vi "my Poisson Random.vi"(6 "seed (-1)":i32=-1, 10 "lambda":dbl=1.0, 11 "samples (1)":i32=1) -> (0 "error":i32, 3 "Poisson random data":i32[](array[numeric]))   [LabVIEW 2021, in "Math.lvlib"]
uses:
  Math.lvlib
  <vilib>/gmath/statdist.llb/st_error_code.ctl
  <vilib>/gmath/statdist.llb/Uniform Random.vi
  <vilib>/gmath/NI_Gmath.lvlib
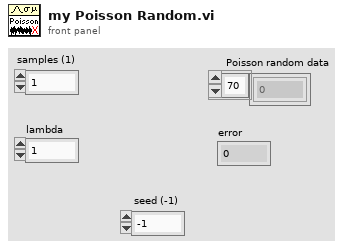
[diagram p1: front panel]
types:
  T1 = typedef "NI_Gmath.lvlib/st_error_code.ctl" = i32
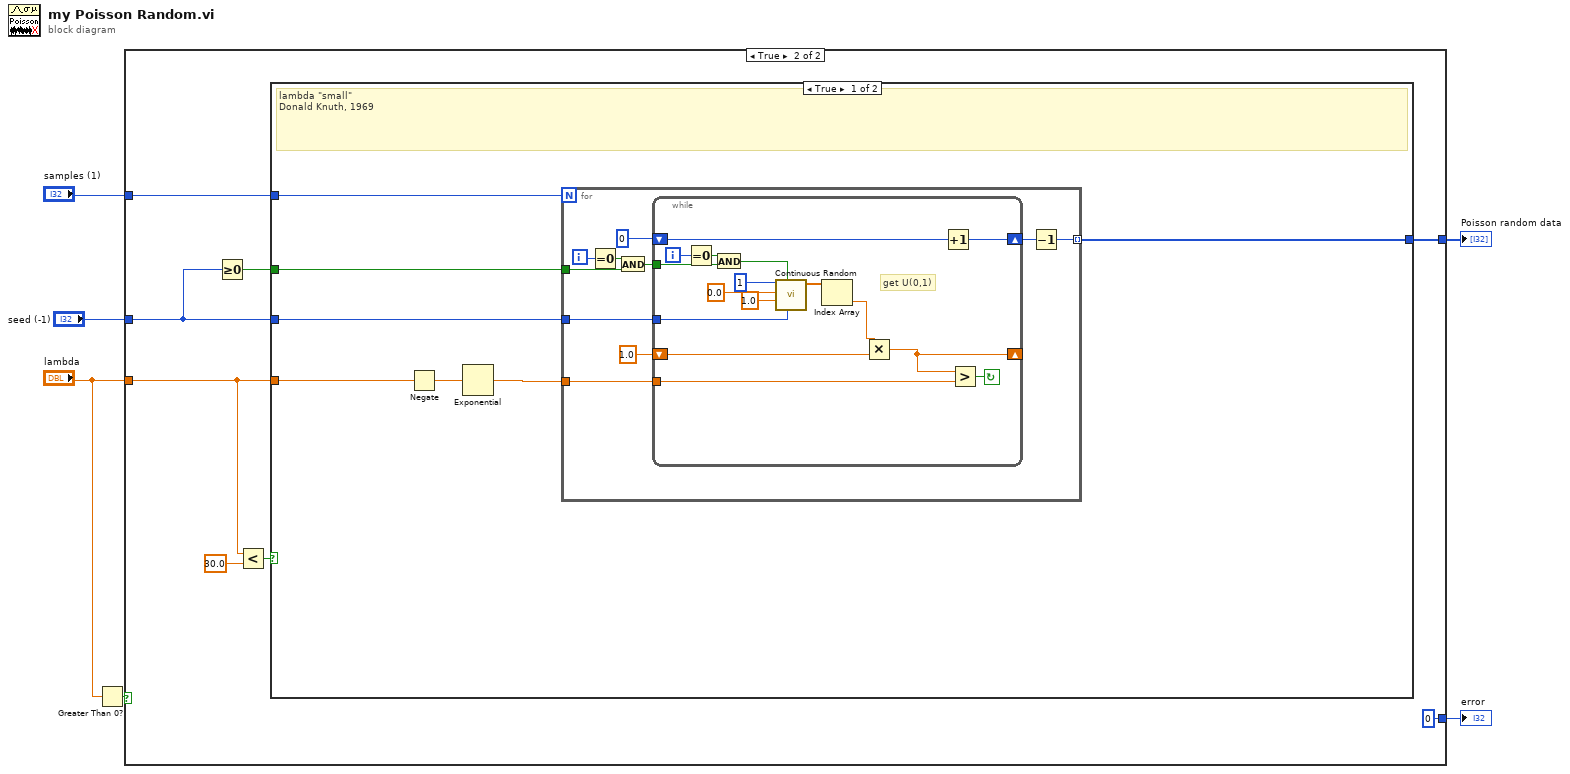
[diagram p0: block diagram]
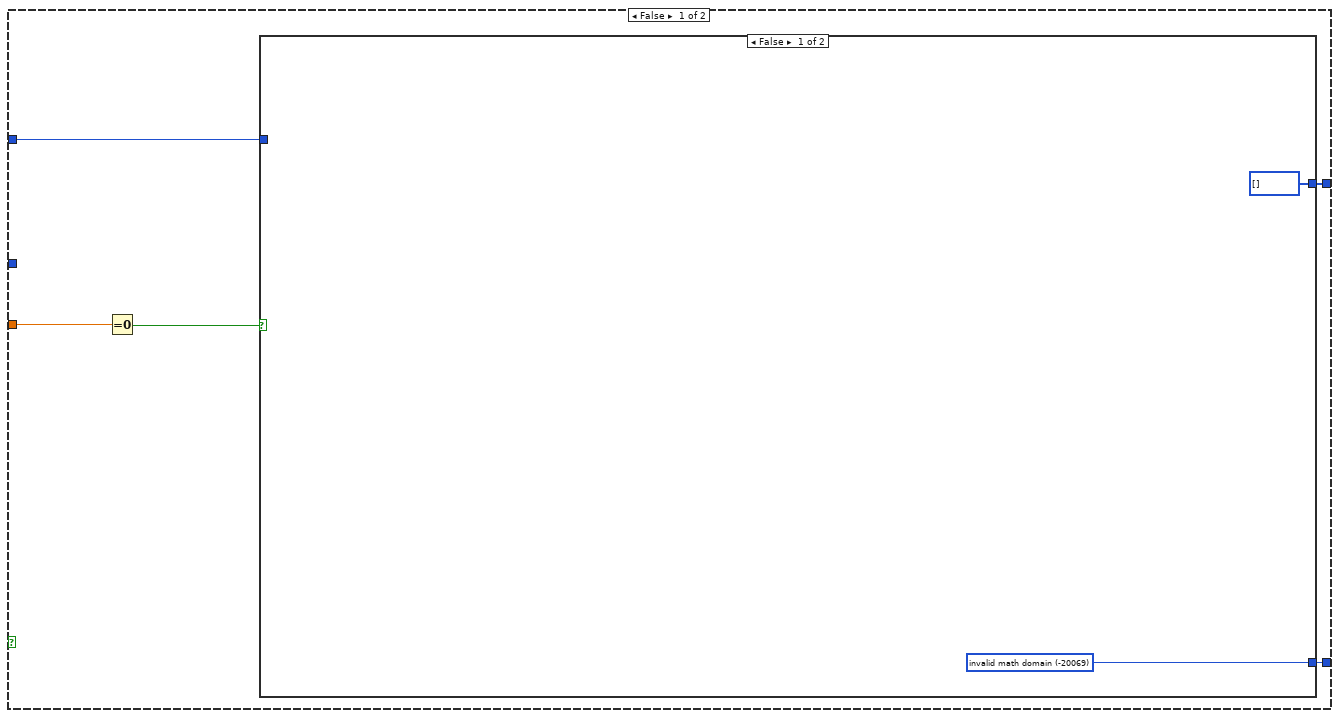
[diagram p2: hidden frame]
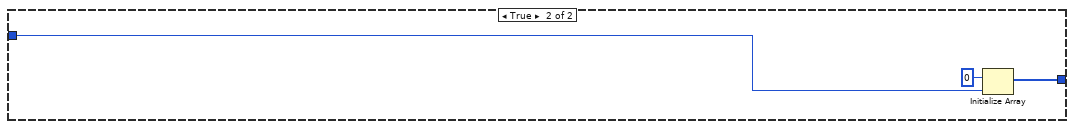
[diagram p3: hidden frame]
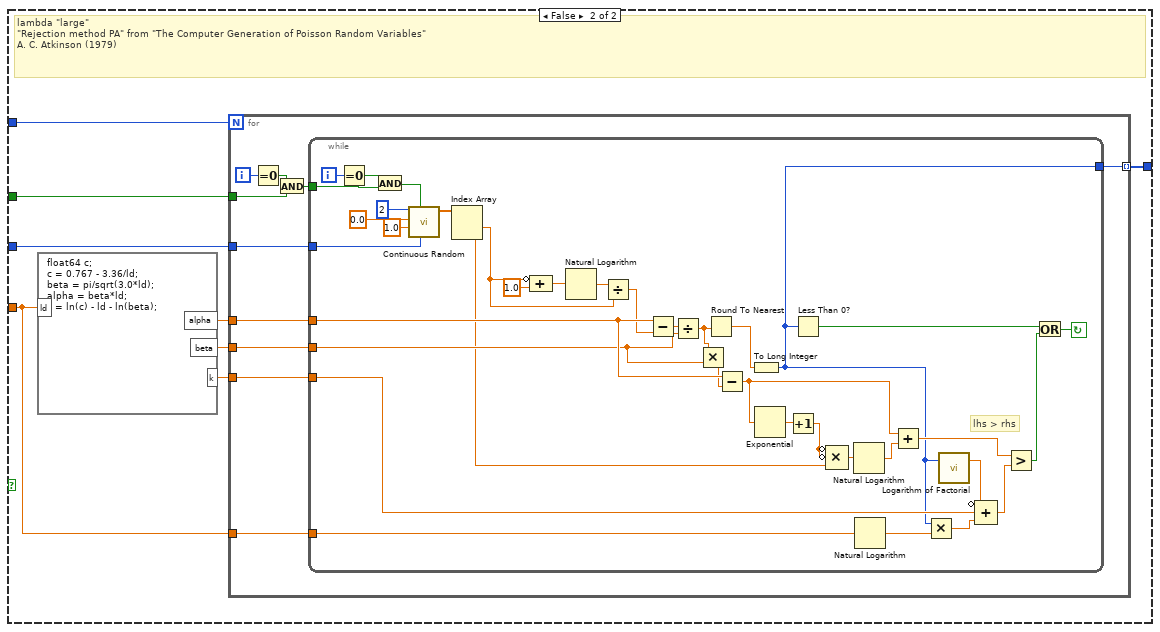
[diagram p4: hidden frame]
diagram:
  n1 = Greater Than 0?(x="lambda") -> (x > 0?=w6:bool)
  n2 = case shown="True" w6 {
    tunnel: [w11 w23] -> w3
    tunnel: "lambda" -> [w9 w19]
    tunnel: [w10 0 ("invalid math domain")] -> w2
    tunnel: "samples (1)" -> [w7 w22]
    tunnel: "seed (-1)" -> [_ w18]
    frame False {
      n3 = Equal To 0?(x=w9) -> (x = 0?=w8:bool)
      n4 = case shown="False" w8 {
        tunnel: [i32[] [] w16] -> w11
        tunnel: [w12 _] -> w10
        tunnel: w7 -> [_ w15]
        frame False {
          w12 = T1 -20069 items=["invalid math domain"=-20069, "Fourier interpolation size m >= n"=-20070, "empty array"=-20003] ("stat interp error code")
        }
        frame True {
          n5 = Initialize Array(0 ("element"), w15) -> (w16:i32[])
        }
      }
    }
    frame True {
      n6 = Greater Or Equal To 0?(x=w18) -> (x >= 0?=w17:bool)
      n7 = Less?(x=w19, y=30.0) -> (x < y?=w21:bool)
      n8 = case shown="True" w21 {
        tunnel: w19 -> [w31 w61]
        tunnel: [w28 w60] -> w23
        tunnel: w22 -> [w27 w65]
        tunnel: w18 -> [w26 w59]
        tunnel: w17 -> [w25 w58]
        frame True {
          # "lambda \"small\"\nDonald Knuth, 1969"
          n9 = Negate(x=w31) -> (-x=w30:dbl)
          n10 = Exponential(1:w30) -> (0:w29:dbl)
          n11 = for {
            N: w27 -> [_]
            tunnel: w29 -> [w40]
            tunnel: [w38] -> w28 mode=indexing
            tunnel: w26 -> [w36]
            tunnel: w25 -> [w34]
            i -> [w32]
            n12 = Equal To 0?(x=w32) -> (x = 0?=w35:bool)
            n13 = And(x=w35, y=w34) -> (x .and. y?=w33:bool)
            n14 = while {
              shift-right: [w56] -> w39
              shift-left: 0 -> [w57]
              tunnel: w40 -> [w55]
              shift-right: [w52] -> _
              shift-left: 1.0 -> [w53]
              tunnel: w36 -> [w46]
              tunnel: w33 -> [w44]
              i -> [w42]
              stop <- w54 continue-if-true
              # "get U(0,1)"
              n15 = Equal To 0?(x=w42) -> (x = 0?=w45:bool)
              n16 = And(x=w45, y=w44) -> (x .and. y?=w43:bool)
              n17 = call-poly <vilib>:"Continuous Random.vi"("seed"=w46, "reset"=w43, "xmax"=1.0, "xmin"=0.0, "samples"=1) -> ("uniform random data"=w51:dbl[])  [unwired: 5 in, 1 out]
              n18 = Index Array(array=w51) -> (element=w47:dbl)  [unwired: 1 in]
              n19 = Multiply(x=w47, y=w53) -> (x*y=w52:dbl)
              n20 = Increment(x=w57) -> (x+1=w56:i32)
              n21 = Greater?(x=w52, y=w55) -> (0:w54:bool)
            }
            n22 = Decrement(x=w39) -> (x-1=w38:i32)
          }
        }
        frame False {
          # "lambda \"large\"\n\"Rejection method PA\" from \"The Computer Generation of Poisson Random Variables\"\nA. C. Atkinson (1979)"
          n23 = formula code="float64 c;\nc = 0.767 - 3.36/ld;\nbeta = pi/sqrt(3.0*ld);\nalpha = beta*ld;\nk = ln(c) - ld - ln(beta);"("ld"=w61) -> ("k"=w62:dbl, "beta"=w63:dbl, "alpha"=w64:dbl)
          n24 = for {
            N: w65 -> [_]
            tunnel: w64 -> [w75]
            tunnel: w63 -> [w74]
            tunnel: w62 -> [w73]
            tunnel: w61 -> [w72]
            tunnel: [w71] -> w60 mode=indexing
            tunnel: w59 -> [w70]
            tunnel: w58 -> [w67]
            i -> [w68]
            n25 = Equal To 0?(x=w68) -> (x = 0?=w69:bool)
            n26 = And(x=w69, y=w67) -> (x .and. y?=w66:bool)
            n27 = while {
              tunnel: w75 -> [w110]
              tunnel: w74 -> [w91]
              tunnel: w73 -> [w100]
              tunnel: w72 -> [w103]
              tunnel: [w94] -> w71
              tunnel: w70 -> [w80]
              tunnel: w66 -> [w79]
              i -> [w77]
              stop <- w111 continue-if-true
              # "lhs > rhs"
              n28 = Equal To 0?(x=w77) -> (x = 0?=w76:bool)
              n29 = And(x=w76, y=w79) -> (x .and. y?=w78:bool)
              n30 = call-poly <vilib>:"Continuous Random.vi"("seed"=w80, "reset"=w78, "xmax"=1.0, "xmin"=0.0, "samples"=2) -> ("uniform random data"=w83:dbl[])  [unwired: 5 in, 1 out]
              n31 = Index Array(array=w83) -> (element #1=w82:dbl, element #2=w81:dbl)  [unwired: 2 in]
              n32 = Compound Arithmetic op=ADD(invert w82, 1.0 ("value")) -> (w89:dbl)
              n33 = Natural Logarithm(1:w89) -> (0:w88:dbl)
              n34 = Divide(x=w88, y=w82) -> (x/y=w87:dbl)
              n35 = Subtract(x=w110, y=w87) -> (x-y=w93:dbl)
              n36 = Divide(x=w93, y=w91) -> (x/y=w92:dbl)
              n37 = Multiply(x=w92, y=w91) -> (x*y=w109:dbl)
              n38 = Round To Nearest(number=w92) -> (nearest integer value=w95:dbl)
              n39 = Subtract(x=w110, y=w109) -> (x-y=w105:dbl)
              n40 = To Long Integer(number=w95) -> (32bit integer=w94:i32)
              n41 = Exponential(1:w105) -> (0:w108:dbl)
              n42 = Increment(x=w108) -> (x+1=w107:dbl)
              n43 = Less Than 0?(x=w94) -> (x < 0?=w112:bool)
              n44 = Compound Arithmetic op=MULTIPLY(invert w107, invert w107, w81) -> (w106:dbl)
              n45 = Natural Logarithm(1:w106) -> (0:w104:dbl)
              n46 = Natural Logarithm(1:w103) -> (0:w102:dbl)
              n47 = Add(x=w105, y=w104) -> (x+y=w97:dbl)
              n48 = Multiply(x=w94, y=w102) -> (x*y=w101:dbl)
              n49 = call <vilib>:"Logarithm of Factorial.vi"("n"=w94) -> ("ln(n!)"=w99:dbl)  [unwired: 2 in]
              n50 = Compound Arithmetic op=ADD(invert w99, w100, w101) -> (w98:dbl)
              n51 = Greater?(x=w97, y=w98) -> (0:w96:bool)
              n52 = Or(x=w112, y=w96) -> (x .or. y?=w111:bool)
            }
          }
        }
      }
    }
  }
  "error" <- w2
  "Poisson random data" <- w3
